vi "Update Position.vi"(0 "PC Bus Address":u32=832 format="%.0x") -> (1 "x mm":dbl, 2 "y mm":dbl)   [LabVIEW 2022 SP3]
uses:
  -MotionRoutines/MotionGlobals.vi
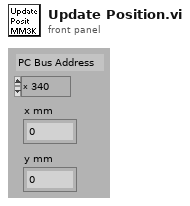
[diagram p1: front panel]
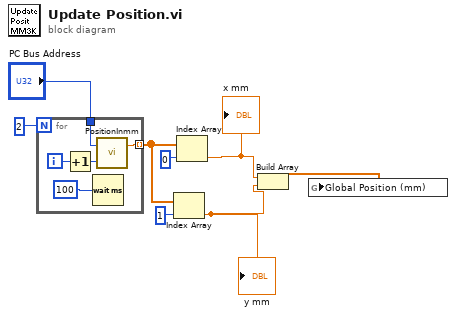
[diagram p0: block diagram]
diagram:
  n1 = for {
    N: 2 -> [_]
    tunnel: [w11] -> w8 mode=indexing
    tunnel: "PC Bus Address" -> [w9]
    i -> [w13]
    n2 = Increment(x=w13) -> (x+1=w12:i32)
    n3 = Wait (ms)(milliseconds to wait=100) -> ()  [unwired: 1 out]
    n4 = call "PositionInmm.vi"("Axis"=w12, "PC Bus Address"=w9) -> ("postion in mm"=w11:dbl)  [unwired: 1 out]
  }
  n5 = Index Array(array=w8, index=1 ("Axis")) -> (element=w2:dbl)
  "y mm" <- w2
  n6 = Index Array(array=w8, index=0 ("Index")) -> (element=w3:dbl)
  "x mm" <- w3
  n7 = Build Array(w3, w2) -> (w1:dbl[])
  n8 = global write "MotionGlobals.vi" "Global Position (mm)"(w1) -> ()
